vi "Agilent VNA Set Instrument Mode.vi"(7 "Agilent VNA":T2, 8 "error in (no error)":errorcluster, 10 "Instrument Mode":T1=enum."NA", 11 "VISA Resource Name":refnum<visa-resource-name>) -> (0 "error out":errorcluster, 3 "dup VISA Resource Name":refnum<visa-resource-name>)   [LabVIEW 2011]
doc: "This VI for the HP8753B Network Analyzers reads the stimulus values. Except when performing log sweeps and freq list sweeps, this VI uses the start and stop values and the number of points to calcuate the stimulus values."
uses:
  TypeDefs/Agilent VNA Instrument Info.ctl
  TypeDefs/Agilent VNA Instrument Mode.ctl
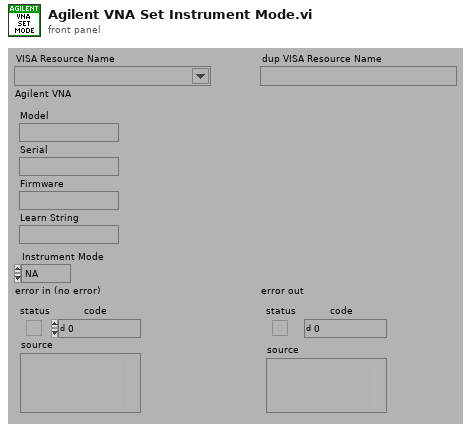
[diagram p1: front panel]
types:
  T1 = typedef "Agilent VNA Instrument Mode.ctl" = enum16{"CAT", "NA", "SA", "Power Meter", "VVM"}
  T2 = typedef "Agilent VNA Instrument Info.ctl" = cluster{"Model":string, "Serial":string, "Firmware":string, "Learn String":string}
  T3 = typedef "Agilent VNA Model.ctl" = enum16{"Not Supported", "8510X", "8719X", "8720X", "8722X", "8753X", "ENA", "PNA", "Field Fox"}
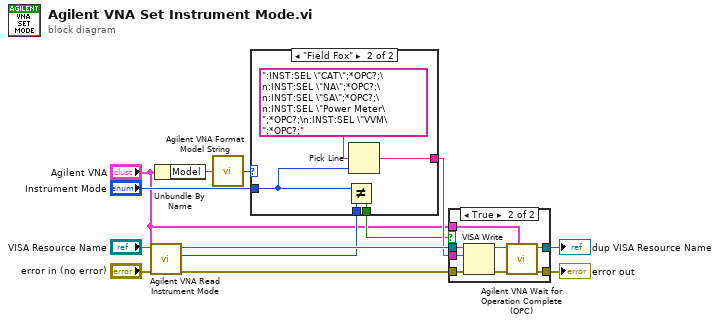
[diagram p0: block diagram]
diagram:
  n1 = call "Agilent VNA Read Instrument Mode.vi"("Agilent VNA"="Agilent VNA", "error in (no error)"="error in (no error)", "VISA Resource Name"="VISA Resource Name") -> ("error out"=w12:errorcluster, "Instrument Mode"=w4:T1, "dup VISA Resource Name"=w13:refnum<visa-resource-name>)  [unwired: 6 in]
  n2 = Unbundle By Name("Agilent VNA") -> ("Model"=w2:string)
  n3 = call "Agilent VNA Format Model String.vi"("Model"=w2) -> ("Model"=w11:T3)
  n4 = case shown="\"Field Fox\"" w11 {
    tunnel: [_ w17] -> w6
    tunnel: "Instrument Mode" -> [_ w16]
    tunnel: w4 -> [_ w15]
    tunnel: [_ w14] -> w3
    frame "Not Supported".."PNA" {
    }
    frame "Field Fox" {
      n5 = Not Equal?(x=w16, y=w15) -> (x != y?=w14:bool)
      n6 = Pick Line(multi-line string=":INST:SEL \"CAT\";*OPC?;\n:INST:SEL \"NA\";*OPC?;\n:INST:SEL \"SA\";*OPC?;\n:INST:SEL \"Power Meter\";*OPC?;\n:INST:SEL \"VVM\";*OPC?;", line index=w16) -> (output string=w17:string)  [unwired: 1 out]
    }
  }
  n7 = case shown="True" w3 {
    tunnel: [w19 w22] -> w7
    tunnel: [w20 w23] -> w8
    tunnel: w6 -> [_ w28]
    tunnel: w13 -> [w20 w27]
    tunnel: w12 -> [w19 w26]
    tunnel: "Agilent VNA" -> [_ w21]
    frame False {
    }
    frame True {
      n8 = VISA Write(VISA resource name=w27, write buffer=w28, error in (no error)=w26) -> (VISA resource name out=w24:refnum<visa-resource-name>, error out=w25:errorcluster)  [unwired: 1 out]
      n9 = call "Agilent VNA Wait for Operation Complete (OPC).vi"("Agilent VNA"=w21, "error in (no error)"=w25, "VISA Resource Name"=w24) -> ("error out"=w22:errorcluster, "dup VISA Resource Name"=w23:refnum<visa-resource-name>)  [unwired: 7 in]
    }
  }
  "dup VISA Resource Name" <- w8
  "error out" <- w7
